vi "Demo - Simple Use.vi"() -> ()   [LabVIEW 2013, in "GOLPI library.lvlib"]
doc: "Very simple demonstration of use of the GOLPI library."
uses:
  GOLPI library.lvlib
panel:
  in  "command":string="sin(3)\n\n"
  out "GNU Octave version":string
  out "exit code":i32
  out "error out":errorcluster
  out "read buffer":string
  in  "Octave binary directory":path=path "C:/Program Files/Octave-3.6.2/bin"
  in  "Working directory":path=path "C:/"
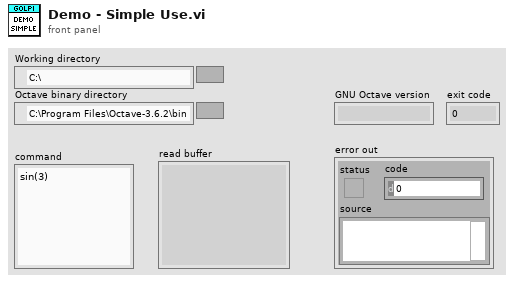
[diagram p1: front panel]
types:
  T1 = typedef "GOLPI library.lvlib/GOLPI reference Type Def.ctl" = cluster{"pipe handle":T2, "fast read timeout [ms]":u32, "fast read settle time [ms]":u32, "fast read to multiple [ms]":u32, "max elements per input line":u32}
  T2 = typedef "LV Process.lvlibp/Pipe Handle.ctl" = cluster{"lv_proc.dll file path":path, "process instance handle":u32[]}
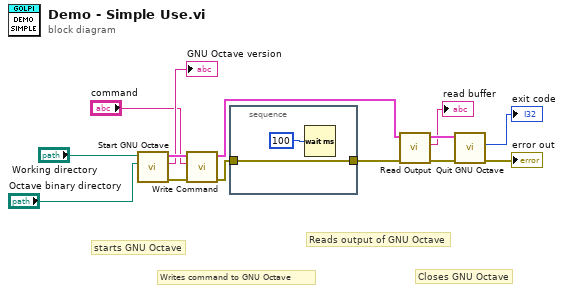
[diagram p0: block diagram]
diagram:
  # "Closes GNU Octave"
  # "Reads output of GNU Octave"
  # "Writes command to GNU Octave"
  # "starts GNU Octave"
  n1 = call "Start GNU Octave.vi"("Octave binary directory"="Octave binary directory", "Working directory"="Working directory") -> ("error out"=w9:errorcluster, "GNU Octave version"=→"GNU Octave version":string, "GOLPI ref. out"=w12:T1)  [unwired: 6 in, 1 out]
  n2 = call "Write Command.vi"("error in"=w9, "command"="command", "GOLPI ref. in"=w12) -> ("error out"=w8:errorcluster, "GOLPI ref. out"=w11:T1)  [unwired: 7 in]
  n3 = stacked-sequence {
    tunnel: [w15] -> w7
    tunnel: w8 -> [w15]
    frame #0 {
      n4 = Wait (ms)(milliseconds to wait=u32 100) -> ()  [unwired: 1 out]
    }
  }
  n5 = call "Read Output.vi"("error in"=w7, "GOLPI ref. in"=w11) -> ("error out"=w5:errorcluster, "read buffer"=→"read buffer":string, "GOLPI ref. out"=w10:T1)  [unwired: 6 in, 1 out]
  n6 = call "Quit GNU Octave.vi"("error in"=w5, "GOLPI ref. in"=w10) -> ("error out"=→"error out":errorcluster, "exit code"=→"exit code":i32)  [unwired: 8 in]
